vi "CheckStartup.vi"(0 "error in":errorcluster, 1 "Get exe":bool, 2 "Load exe":bool, 3 "connection ID in":refnum<k5>, 5 "Load latest":bool) -> (4 "startup there?":bool, 6 "error out":errorcluster, 7 "Good Reply?":bool, 8 "startup dir":string, 9 "connection ID out":refnum<k5>)   [LabVIEW 2012]
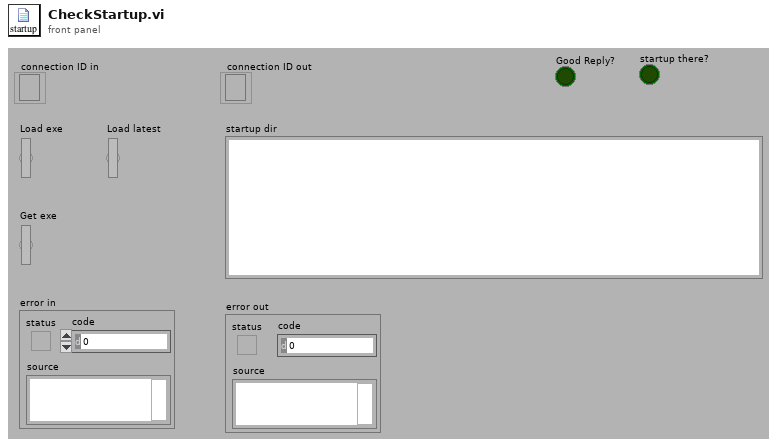
[diagram p1: front panel]
types:
  T1 = enum16{"big-endian, network order", "native, host order", "little-endian"}
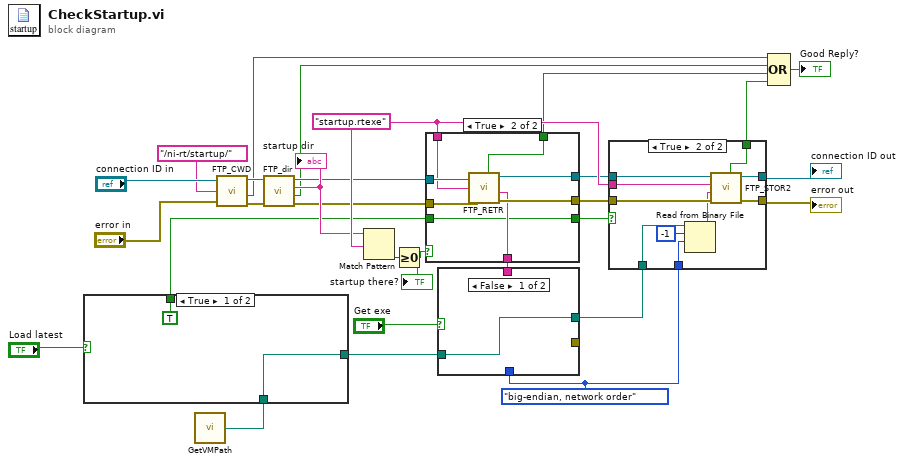
[diagram p0: block diagram]
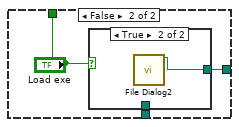
[diagram p2: hidden frame]
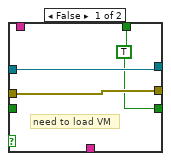
[diagram p4: hidden frame]
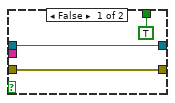
[diagram p5: hidden frame]
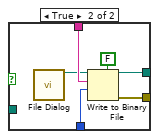
[diagram p6: hidden frame]
diagram:
  w25 = T1."big-endian, network order" ("byte order (0:big-endian, network order)")
  w27 = "startup.rtexe" ("Remote Path")
  n1 = call <userlib>:"GetVMPath.vi"() -> ("appended path"=w4:path)  [unwired: 1 out]
  n2 = case shown="True" "Load latest" {
    tunnel: [w31 w34] -> w5
    tunnel: w4 -> [w31 w33]
    tunnel: [TRUE ("Load exe") "Load exe"] -> w2
    frame True {
    }
    frame False {
      n3 = case shown="True" "Load exe" {
        tunnel: [w35 w36] -> w34
        tunnel: w33 -> [w35 _]
        frame False {
        }
        frame True {
          n4 = call "File Dialog2"() -> ("selected path"=w36:path)  [unwired: 12 in, 3 out]
        }
      }
    }
  }
  n5 = call <userlib>:"FTP_CWD.vi"("connection ID"="connection ID in", "path"="/ni-rt/startup/", "error in"="error in") -> ("connection ID out"=w15:refnum<k5>, "Good Reply?"=w13:bool, "error out"=w16:errorcluster)  [unwired: 1 out]
  n6 = call <userlib>:"FTP_dir.vi"("connection ID"=w15, "error in"=w16) -> ("connection ID out"=w17:refnum<k5>, "reply string"=w26:string, "Good Reply?"=w12:bool, "error out"=w18:errorcluster)  [unwired: 1 out]
  "startup dir" <- w26
  n7 = Match Pattern(string=w26, regular expression=w27) -> (offset past match=w8:i32)  [unwired: 1 in, 3 out]
  n8 = Greater Or Equal To 0?(x=w8) -> (x >= 0?=w7:bool)
  "startup there?" <- w7
  n9 = case shown="True" w7 {
    tunnel: w17 -> [w39 w47]
    tunnel: w18 -> [w38 w46]
    tunnel: [w39 w45] -> w20
    tunnel: w27 -> [_ w44]
    tunnel: [w38 w43] -> w21
    tunnel: [_ w42] -> w24
    tunnel: [w37 w41] -> w11
    tunnel: [w37 w40] -> w3
    tunnel: w2 -> [_ w40]
    frame False {
      w37 = TRUE ("Load exe")
      # "need to load VM"
    }
    frame True {
      n10 = call <userlib>:"FTP_RETR.vi"("connection ID"=w47, "Remote Path"=w44, "error in"=w46) -> ("connection ID out"=w45:refnum<k5>, "vi"=w42:string, "error out"=w43:errorcluster, "Good Reply?"=w41:bool)  [unwired: 1 out]
    }
  }
  n11 = case shown="False" "Get exe" {
    tunnel: w24 -> [_ w53]
    tunnel: w25 -> [_ w51]
    tunnel: [_ w50] -> _
    tunnel: [w48 w49] -> w6
    tunnel: w5 -> [w48 _]
    frame False {
    }
    frame True {
      n12 = call "File Dialog"() -> ("selected path"=w49:path)  [unwired: 12 in, 3 out]
      n13 = Write to Binary File(file (use dialog)=w49, data=w53, 5:FALSE ("prepend array or string size? (T)"), 9:w51) -> (error out=w50:errorcluster)  [unwired: 2 in, 2 out]
    }
  }
  n14 = case shown="True" w3 {
    tunnel: w20 -> [w56 w66]
    tunnel: w27 -> [_ w65]
    tunnel: w21 -> [w55 w64]
    tunnel: [w55 w63] -> w22
    tunnel: [w56 w62] -> w23
    tunnel: w25 -> [_ w59]
    tunnel: [TRUE ("Good Reply?") w58] -> w10
    tunnel: w6 -> [_ w57]
    frame False {
    }
    frame True {
      n15 = Read from Binary File(9:w59, 10:-1 ("count (1)"), 11:w57) -> (2:w60:string)  [unwired: 3 in, 3 out]
      n16 = call <userlib>:"FTP_STOR2.vi"("error in"=w64, "File to send"=w60, "Remote Path"=w65, "connection ID"=w66) -> ("Good Reply?"=w58:bool, "error out"=w63:errorcluster, "connection ID out"=w62:refnum<k5>)  [unwired: 1 in, 1 out]
    }
  }
  "connection ID out" <- w23
  "error out" <- w22
  n17 = Compound Arithmetic op=OR(w13, w12, w11, w10) -> (→"Good Reply?":bool)
